vi "Get Next Sequential Step.vi"(8 "error in (no error)":errorcluster, 10 "Current Step":i32, 11 "Output Sequencer in":refnum<class "Output Sequencer.lvclass">) -> (0 "error out":errorcluster, 1 "Next Cycle?":bool, 2 "Next Step":i32, 3 "Output Sequencer out":refnum<class "Output Sequencer.lvclass">, 4 "Number of Steps":i32)   [LabVIEW 2020, in "Output Sequencer.lvlib" / "Output Sequencer.lvclass"]
uses:
  Output Sequencer.lvclass
  Output Sequencer.lvclass/Output Sequencer.ctl
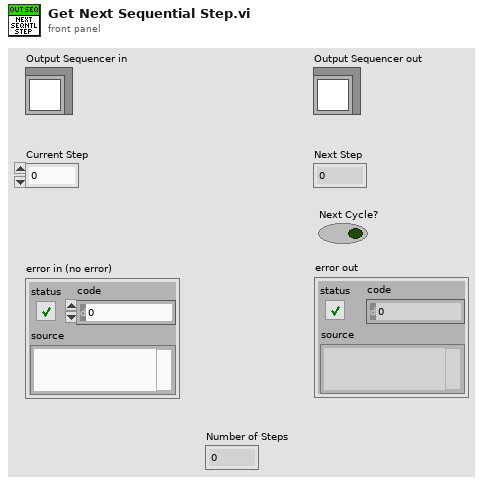
[diagram p1: front panel]
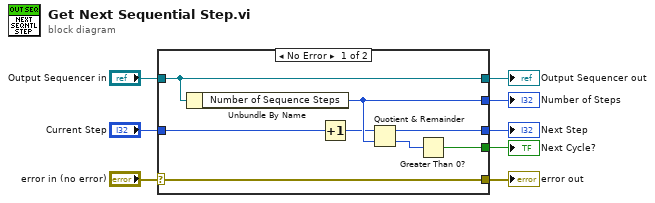
[diagram p0: block diagram]
diagram:
  n1 = case shown="No Error" "error in (no error)" {
    selector: "error in (no error)" -> [w10 w18]
    tunnel: [w16 _] -> w8
    tunnel: [w15 _] -> w7
    tunnel: [w14 _] -> w6
    tunnel: "Current Step" -> [w13 _]
    tunnel: "Output Sequencer in" -> [w9 w17]
    tunnel: [w10 w18] -> w2
    tunnel: [w9 w17] -> w1
    frame No Error {
      n2 = Unbundle By Name(w9) -> ("Number of Sequence Steps"=w14:i32)
      n3 = Increment(x=w13) -> (x+1=w12:i32)
      n4 = Quotient & Remainder(x=w12, y=w14) -> (x-y*floor(x/y)=w15:i32, floor(x/y)=w11:i32)
      n5 = Greater Than 0?(x=w11) -> (x > 0?=w16:bool)
    }
    frame Error {
    }
  }
  "Next Cycle?" <- w8
  "Next Step" <- w7
  "Number of Steps" <- w6
  "Output Sequencer out" <- w1
  "error out" <- w2
